vi "deltaT.vi"() -> ()   [LabVIEW 2016]
panel:
  out "delta t":u32
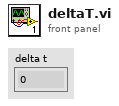
[diagram p1: front panel]
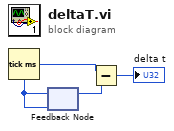
[diagram p0: block diagram]
diagram:
  n1 = Tick Count (ms)() -> (millisecond timer value=w3:u32)
  n2 = feedback-in #1(w3) -> ()
  n3 = feedback #1(w3) -> (w2:u32)
  n4 = Subtract(x=w3, y=w2) -> (x-y=→"delta t":u32)
